vi "GetSpeed.vi"(5 "Max Window":dbl=1800.0 format="%.4f", 7 "Min Window":dbl=300.0 format="%.4f", 8 "error in (no error)":errorcluster, 9 "Y":dbl[](array[numeric]), 10 "FFT Waveform":waveform(dbl), 11 "comm seg":dbl=2.0) -> (0 "error out":errorcluster, 3 "Speed":dbl)   [LabVIEW 2013]
uses:
  <vilib>/addons/Spectral Measurements Toolset/LVSupport/SMT Zoom Power Spectrum (WDT).vi
  <vilib>/addons/Spectral Measurements Toolset/niSMT.lvlib
panel:
  out "Waveform Graph 2":dbl[](graph)
  in  "update?":bool
  out "Waveform Graph":dbl[](graph)
  out "peaks":cluster{"frequency":dbl, "value":dbl}[](array[cluster]) {"value" format="%.2f"; "frequency" format="%.2f"}
  in  "advanced settings":T1={"window"=enum."7 Term B-Harris", "spectral lines"=-1, "effective band specification"={"fl"=0.0, "fh"=0.5}, "RBW definition"=enum."3dB"} {"effective band specification"."fh" format="%.2f"; "effective band specification"."fl" format="%.2f"}
  in  "spectrum settings":T2={"center frequency"=12000000.0, "span"=5000000.0, "resolution bandwidth"=-1.0} {"resolution bandwidth" format="%.2p"; "center frequency" format="%.2p"; "span" format="%.2p"}
  in  "averaging parameters":T3={"averaging type"=enum."no averaging", "averaging settings"={"weighting type"=enum."exponential", "weighting settings"={"size"=1.0, "linear weighting mode"=enum."moving average"}}}
  in  "peak search settings":T4={"single/multiple"=enum."Single Max Peak", "threshold"=0.01} {"threshold" format="%.2f"}
  in  "unit conversion settings":T5={"units"=enum."V", "peak scaling"=enum."rms", "psd?"=FALSE, "impedance(ohm)"=50.0} {"impedance(ohm)" format="%.2f"}
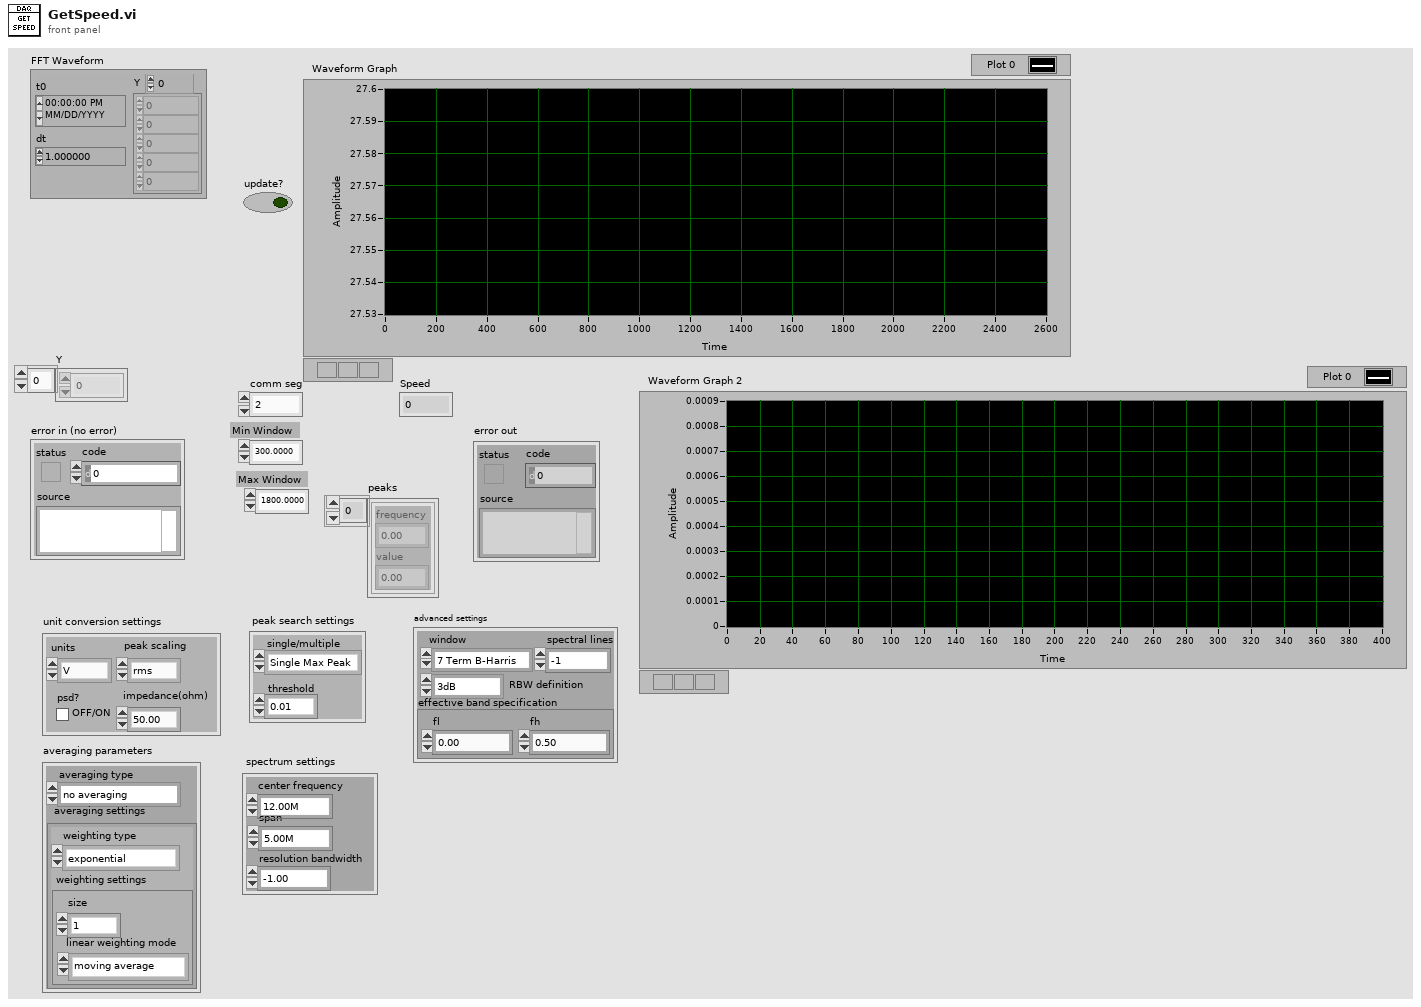
[diagram p1: front panel]
types:
  T1 = cluster{"window":enum16{"None ", "Hanning", "Hamming", "Blackman-Harris", "Exact Blackman", "Blackman", "Flat Top", "4 Term B-Harris ", "7 Term B-Harris", "Low Sidelobe"}, "spectral lines":i32, "effective band specification":cluster{"fl":dbl, "fh":dbl}, "RBW definition":enum16{"3dB", "6dB", "ENBW", "bin width"}}
  T2 = cluster{"center frequency":dbl, "span":dbl, "resolution bandwidth":dbl}
  T3 = cluster{"averaging type":enum16{"no averaging", "vector averaging", "RMS averaging", "peak hold"}, "averaging settings":cluster{"weighting type":enum16{"linear", "exponential"}, "weighting settings":cluster{"size":dbl, "linear weighting mode":enum16{"one shot", "auto restart one shot", "moving average", "continuous"}}}}
  T4 = cluster{"single/multiple":enum16{"Multiple Peaks", "Single Max Peak"}, "threshold":dbl}
  T5 = cluster{"units":enum16{"V", "V^2", "W", "dBm", "dBW", "dBV", "dBmV", "dBuV"}, "peak scaling":enum16{"rms", "pk"}, "psd?":bool, "impedance(ohm)":dbl}
  T6 = cluster{"type":enum16{"real", "complex modulated"}, "frequency shift":dbl}
  T7 = typedef "niSMT.lvlib/SMT zoom settings.ctl" = cluster{"zoom FFT settings":T8, "frequency shift":dbl, "data format":enum16{"real", "complex modulated (array)", "complex modulated (interleaved)"}}
  T8 = typedef "NI_MAPro.lvlib/ma_sml_ND Zoom FFT Settings.ctl" = cluster{"zoom settings":cluster{"center frequency":dbl, "zoom":i32, "trim":dbl}, "FFT settings":cluster{"window":u16, "FFT size":i32}}
  T9 = typedef "NI_MAPro.lvlib/ma_sml_Spectral Info.ctl" = cluster{"spectrum type":enum16{"FFT Spectrum [complex]", "Amplitude [Magnitude]", "Power [Magnitude^2]", "Cross Spectrum [complex]", "Frequency Response [Complex]"}, "linear/dB":enum16{"linear", "dB"}, "window":u16, "window size":i32, "FFT size":i32}
  T10 = typedef "NI_MAPro.lvlib/ma_sml_Spectrum Cluster (real).ctl" = cluster{"f0":dbl, "df":dbl, "spectrum":dbl[]}
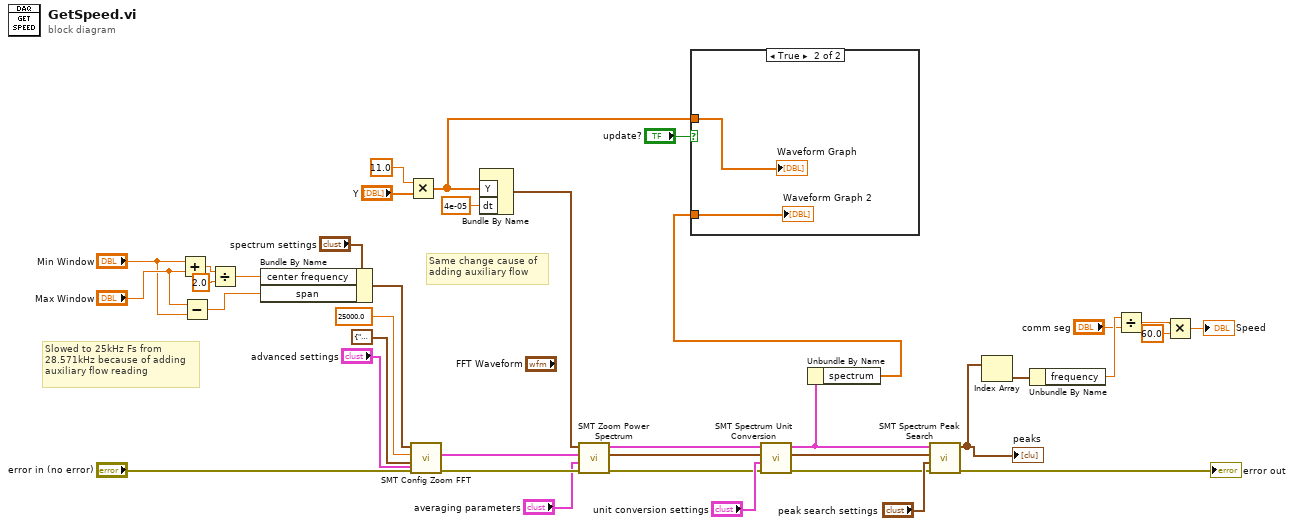
[diagram p0: block diagram]
diagram:
  # "Same change cause of\nadding auxiliary flow"
  # "Slowed to 25kHz Fs from\n28.571kHz because of adding\nauxiliary flow reading"
  n1 = Add(x="Min Window", y="Max Window") -> (x+y=w28:dbl)
  n2 = Subtract(x="Max Window", y="Min Window") -> (x-y=w30:dbl)
  n3 = Divide(x=w28, y=2.0) -> (x/y=w26:dbl)
  n4 = Bundle By Name(cluster="spectrum settings", "center frequency"=w26, "span"=w30) -> (w31:T2)
  n5 = Multiply(x=11.0, y="Y") -> (x*y=w5:dbl[])
  n6 = call <vilib>:"SMT Config Zoom FFT.vi"("advanced settings"="advanced settings", "error in (no error)"="error in (no error)", "input signal settings"=T6 {"type"=enum."real", "frequency shift"=0.0}, "fs"=25000.0, "spectrum settings"=w31) -> ("error out"=w22:errorcluster, "SMT zoom settings"=w21:T7)  [unwired: 3 in, 2 out]
  n7 = Bundle By Name("Y"=w5, "dt"=4e-05) -> (w8:waveform(dbl))  [unwired: 1 in]
  n8 = call-poly <vilib>:"SMT Zoom Power Spectrum.vi"("error in (no error)"=w22, "averaging parameters"="averaging parameters", "SMT zoom settings"=w21, "signal in"=w8) -> ("error out"=w17:errorcluster, "spectral info"=w16:T9, "power spectrum"=w23:T10)  [unwired: 3 in, 2 out]
  n9 = call <vilib>:"SMT Spectrum Unit Conversion.vi"("error in (no error)"=w17, "unit conversion settings"="unit conversion settings", "spectral info in"=w16, "power spectrum"=w23) -> ("error out"=w15:errorcluster, "spectral info out"=w3:T9, "unit converted spectrum"=w2:cluster{"f0":dbl, "df":dbl, "spectrum":dbl[]})  [unwired: 4 in, 1 out]
  n10 = Unbundle By Name(w2) -> ("spectrum"=w1:dbl[])
  n11 = case shown="True" "update?" {
    tunnel: w5 -> [_ w40]
    tunnel: w1 -> [_ w39]
    frame False {
    }
    frame True {
      "Waveform Graph" <- w40
      "Waveform Graph 2" <- w39
    }
  }
  n12 = call <vilib>:"SMT Spectrum Peak Search.vi"("error in (no error)"=w15, "peak search setting"="peak search settings", "spectral info"=w3, "power spectrum"=w2) -> ("error out"=→"error out":errorcluster, "peaks"=w13:cluster{"frequency":dbl, "value":dbl}[])  [unwired: 5 in, 1 out]
  "peaks" <- w13
  n13 = Index Array(array=w13) -> (element=w32:cluster{"frequency":dbl, "value":dbl})  [unwired: 1 in]
  n14 = Unbundle By Name(w32) -> ("frequency"=w14:dbl)
  n15 = Divide(x=w14, y="comm seg") -> (x/y=w33:dbl)
  n16 = Multiply(x=w33, y=60.0) -> (x*y=→"Speed":dbl)
